vi "Message Log Headers.vi"() -> (3 "Message Log Headers":string[](array[string]))   [LabVIEW 2017, in "Message Log.lvclass"]
uses:
  Message Log.lvclass
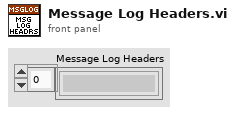
[diagram p1: front panel]
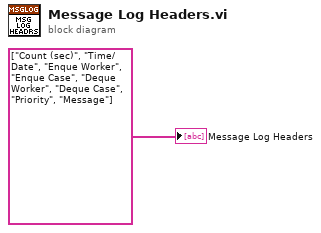
[diagram p0: block diagram]
diagram:
  "Message Log Headers" <- string[] ["Count (sec)", "Time/Date", "Enque Worker", "Enque Case", "Deque Worker", "Deque Case", "Priority", "Message"] ("L10n_item tags 2")
